vi "beginPassToStrikerPlay.vi"(8 "error in (no error)":errorcluster, 10 "Game":refnum<class "Game.lvclass">, 11 "PassToStriker in":refnum<class "PassToStriker.lvclass">) -> (0 "error out":errorcluster, 2 "BeginPassToStriker?":bool, 3 "PassToStriker out":refnum<class "PassToStriker.lvclass">)   [LabVIEW 2020, in "PassToStriker.lvclass"]
uses:
  PassToStriker.lvclass
  Game_class/Game.lvclass
  Utilities_class/Utilities.lvclass
  Team_class/OffensivePlay.ctl
  Game_class/Game.lvclass/Game.ctl
  Team_class/Team.lvclass/Team.ctl
  Referee_class/Referee.lvclass/Referee.ctl
  Referee_class/command_interpreted.ctl
  Game_class/Read Referee.vi
  Referee_class/Read command_interpreted.vi
  Game_class/Read OffensiveTeam.vi
  Team_class/Read RobotRef.vi
  Team_class/Read OffensivePlay.vi
  Ally_class/Ally.lvclass
  Robot_class/Robot.lvclass
  Referee_class/Referee.lvclass
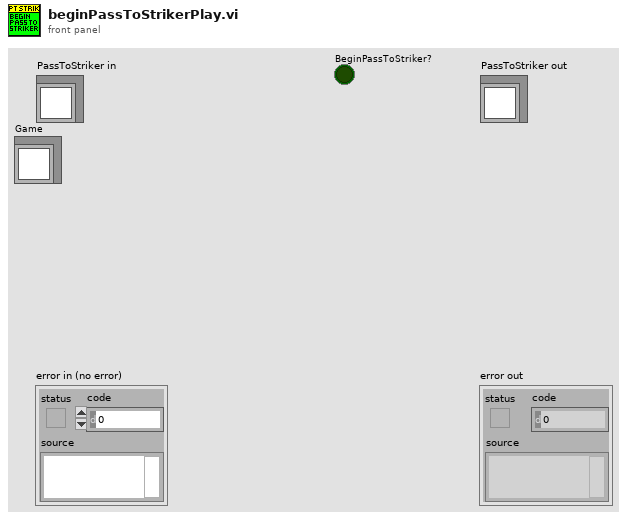
[diagram p1: front panel]
types:
  T1 = typedef "command_interpreted.ctl" = enum16{"Goal Ally", "Goal Enemy", "Ball Placement Enemy", "Ball Placement Ally", "Normal Half Time", "Extra Time  Break", "Extra Half Time", "None", "Post Game", "PKA Normal Start", "Prepare Kickoff Ally", "PKE Normal Start", "Prepare Kickoff Enemy", "Force Start", "Halt", "Timeout", "Prepare Penalty Ally", "Prepare Penalty Enemy", "PPA NormalStart", "PPE Normal Start", "Indirect Free Ally", "Direct Free Enemy", "Direct Free Ally", "Indirect Free Enemy", "Stop"}
  T2 = typedef "OffensivePlay.ctl" = enum16{"ABCPass", "PrepareTriplePass", "TableWithStriker", "TableWith2ndStrikerPlay", "PrepareDoublePass", "PrepareRollToPass", "SimplePass", "PreparePass", "PassToStriker", "BallOutOfField", "PassTo2ndStriker", "StopOffensive", "Prepare Penalty Enemy", "EnemyPossessionAtEnemyField", "EnemyPossesionAtOurField", "TestPlay", "PreparePenaltyAlly", "KickPenaltyAlly", "PrepareKickoffAlly", "PrepareKickoffEnemy", "IndirectEnemy", "DirectEnemy", "PreparePassInGame1", "NormalGame", "DirectKick", "Pass", "Halt", "Timeout", "PassPlay", "PenaltyEnemy"}
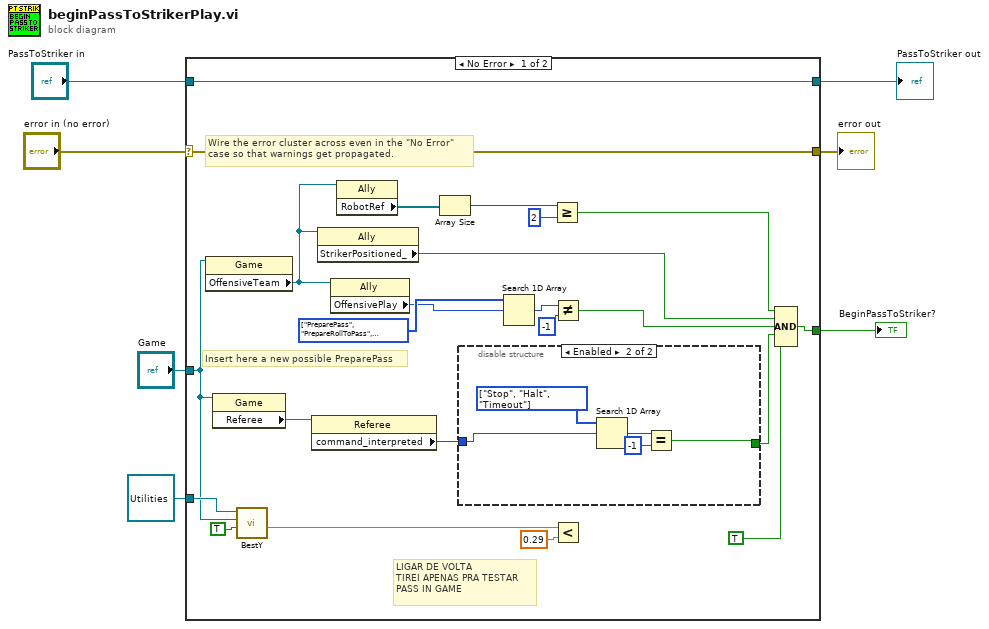
[diagram p0: block diagram]
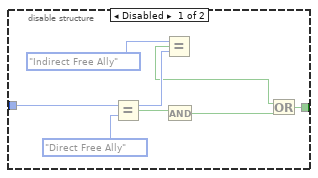
[diagram p2: hidden frame]
diagram:
  n1 = case shown="No Error" "error in (no error)" {
    selector: "error in (no error)" -> [w29 w44]
    tunnel: [w29 w44] -> w6
    tunnel: [w30 w43] -> w4
    tunnel: "PassToStriker in" -> [w30 w43]
    tunnel: "Game" -> [w22 _]
    tunnel: refnum<class "Utilities.lvclass"> refnum ("Utilities.lvclass") -> [w23 _]
    tunnel: [w21 _] -> w1
    frame No Error {
      w13 = T2[] [enum."PreparePass", enum."PrepareRollToPass", enum."PreparePassInGame1"] items=["ABCPass", "PrepareTriplePass", "TableWithStriker", "TableWith2ndStrikerPlay", "PrepareDoublePass", "PrepareRollToPass", "SimplePass", "PreparePass", "PassToStriker", "BallOutOfField", "PassTo2ndStriker", "StopOffensive", "Prepare Penalty Enemy", "EnemyPossessionAtEnemyField", "EnemyPossesionAtOurField", "TestPlay", "PreparePenaltyAlly", "KickPenaltyAlly", "PrepareKickoffAlly", "PrepareKickoffEnemy", "IndirectEnemy", "DirectEnemy", "PreparePassInGame1", "NormalGame", "DirectKick", "Pass", "Halt", "Timeout", "PassPlay", "PenaltyEnemy"] ("Array")
      # "LIGAR DE VOLTA\nTIREI APENAS PRA TESTAR\nPASS IN GAME"
      # "Insert here a new possible PreparePass"
      # "Wire the error cluster across even in the \"No Error\"\ncase so that warnings get propagated."
      n2 = property class="Game"(reference=w22) -> ("OffensiveTeam"=w19:refnum<class "Ally.lvclass">)  [unwired: 1 in, 2 out]
      n3 = property class="Game"(reference=w22) -> ("Referee"=w28:refnum<class "Referee.lvclass">)  [unwired: 1 in, 2 out]
      n4 = call "BestY.vi"("Utilities in"=w23, "Game"=w22, "inimigos"=TRUE) -> ("Gap kick"=w24:dbl)  [unwired: 2 in, 4 out]
      n5 = property class="Referee"(reference=w28) -> ("command_interpreted"=w27:T1)  [unwired: 1 in, 2 out]
      n6 = property class="Ally"(reference=w19) -> ("StrikerPositioned_"=w20:bool)  [unwired: 1 in, 2 out]
      n7 = property class="Ally"(reference=w19) -> ("OffensivePlay"=w12:T2)  [unwired: 1 in, 2 out]
      n8 = property class="Ally"(reference=w19) -> ("RobotRef"=w18:refnum<class "Robot.lvclass">[])  [unwired: 1 in, 2 out]
      n9 = Array Size(array=w18) -> (size(s)=w17:i32)
      n10 = disable-structure shown="Enabled" {
        disable-tunnel: w27 -> [w36 w42]
        disable-tunnel: [w31 w38] -> w14
        frame Disabled {
          n11 = Equal?(x=w36, y=command_interpreted."Direct Free Ally" ("command_interpreted")) -> (x = y?=w34:bool)
          n12 = Equal?(x=command_interpreted."Indirect Free Ally" ("command_interpreted"), y=w36) -> (x = y?=w32:bool)
          n13 = And(x=w34) -> (x .and. y?=w33:bool)  [unwired: 1 in]
          n14 = Or(x=w32, y=w33) -> (x .or. y?=w31:bool)
        }
        frame Enabled {
          w41 = T1[] [enum."Stop", enum."Halt", enum."Timeout"] items=["Goal Ally", "Goal Enemy", "Ball Placement Enemy", "Ball Placement Ally", "Normal Half Time", "Extra Time  Break", "Extra Half Time", "None", "Post Game", "PKA Normal Start", "Prepare Kickoff Ally", "PKE Normal Start", "Prepare Kickoff Enemy", "Force Start", "Halt", "Timeout", "Prepare Penalty Ally", "Prepare Penalty Enemy", "PPA NormalStart", "PPE Normal Start", "Indirect Free Ally", "Direct Free Enemy", "Direct Free Ally", "Indirect Free Enemy", "Stop"] ("1D array")
          n15 = Search 1D Array(1D array=w41, element=w42) -> (index of element=w40:i32)  [unwired: 1 in]
          n16 = Equal?(x=w40, y=-1) -> (x = y?=w38:bool)
        }
      }
      n17 = Search 1D Array(1D array=w13, element=w12) -> (index of element=w11:i32)  [unwired: 1 in]
      n18 = Greater Or Equal?(x=w17, y=2) -> (x >= y?=w15:bool)
      n19 = Not Equal?(x=w11, y=-1) -> (x != y?=w9:bool)
      n20 = Less?(x=w24, y=0.29 ("Gap kick")) -> ()  [unwired: 1 out]
      n21 = Compound Arithmetic op=AND(w15, w20, w9, w14, TRUE) -> (w21:bool)
    }
    frame Error {
    }
  }
  "error out" <- w6
  "PassToStriker out" <- w4
  "BeginPassToStriker?" <- w1
